vi "Name.vi"(11 "Path Data Type in":refnum<class "Path Data Type.lvclass">) -> (2 "String":string="Generic", 3 "Path Data Type (dup)":refnum<class "Path Data Type.lvclass">)   [LabVIEW 2018, in "Path Data Type.lvclass"]
uses:
  Path Data Type.lvclass
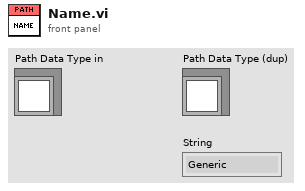
[diagram p1: front panel]
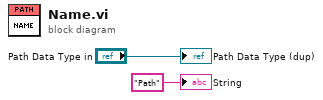
[diagram p0: block diagram]
diagram:
  "Path Data Type (dup)" <- "Path Data Type in"
  "String" <- "Path" ("String")
